vi "CCarga_LVDT_Actuador.vi"() -> ()   [LabVIEW 2015]
uses:
  <vilib>/Utility/file.llb/Read Delimited Spreadsheet (DBL).vi
  variables offset.vi
panel:
  in  "Instrucciones":bool
  out "LVDT RAW":dbl
  out "LVDT":dbl
  out "vector poros":dbl[](array[numeric]) format="%.2f"
  out "C_Poros":dbl
  out "P_Poros":dbl
  out "Poros":dbl
  out "offset 9":dbl
  in  "SAVE":bool
  in  "Tiempo \nMuestreo":dbl=3.0 format="%#_13g"
  out "READ!":bool
  in  "BttActuador":bool
  out "Boolean":bool
  out "offset 8":dbl
  out "offset 7":dbl
  in  "offsets":bool
  out "C_Celda":dbl
  out "C_lvdt":dbl
  out "P_Celda":dbl
  out "P_lvdt":dbl
  out "all rows":dbl[][](array[numeric])
  out "vector carga":dbl[](array[numeric]) format="%.2f"
  out "vector desp":dbl[](array[numeric]) format="%.2f"
  out "Carga":dbl
  in  "Tab Control":enum32{"SENSORES"}(tab)
  out "Waveform Celda de Carga":dynamicdata(graph)
  out "Waveform LVDT":dynamicdata(graph)
  out "LOAD RAW":dbl
  out "Waveform Presión de Poros":dynamicdata(graph)
  out "TIME SEC":dbl[](array[numeric]) format="%.2f"
  out "x/y":dbl
  out "Boolean 2":bool
  out "tiempo [min]":ext
  out "path":path
  in  "stop":bool
  in  "Conect":bool
  in  "Filename":path=path "Ensayo_Dyn_M"
  # "Seg."
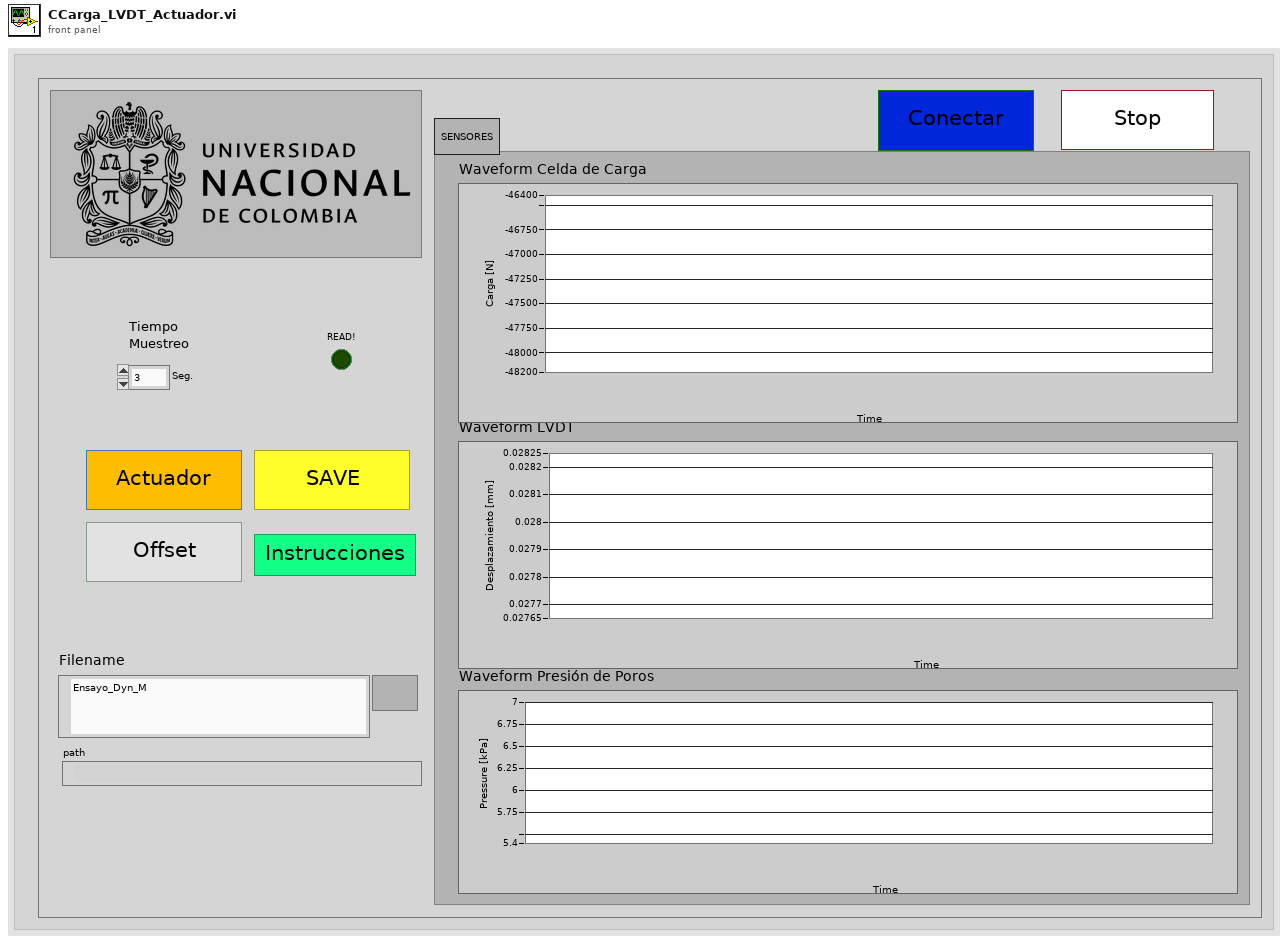
[diagram p1: front panel]
types:
  T1 = enum16{"open", "open or create", "create or replace", "create", "open (read-only)"}
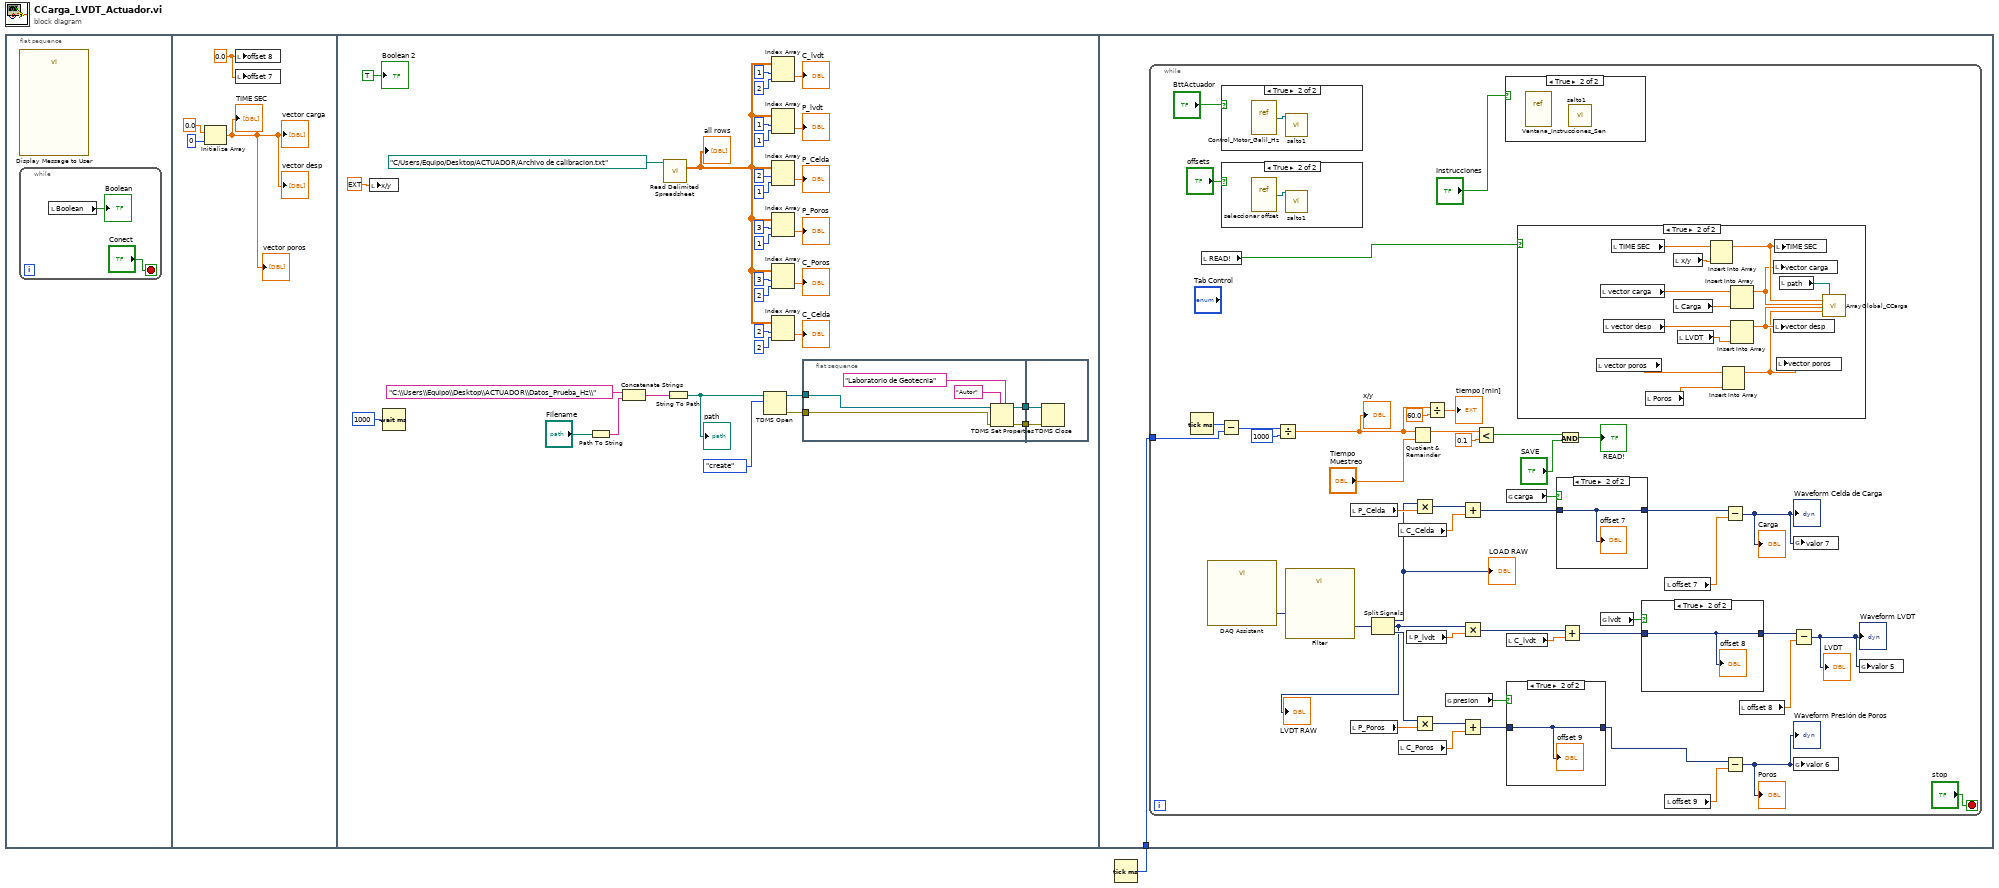
[diagram p0: block diagram]
diagram:
  n1 = flat-sequence {
    tunnel: w1 -> [w49]
    frame #0 {
      n2 = call "Display Message to User"() -> ()  [unwired: 10 in, 2 out]
      n3 = while {
        stop <- "Conect" stop-if-true
        n4 = local read "Boolean"() -> (→"Boolean":bool)
      }
    }
    frame #1 {
      w5 = 0.0
      n5 = Initialize Array(0.0, 0 ("dimension size")) -> (→"TIME SEC" →"vector desp" →"vector carga" →"vector poros":dbl[])
      n6 = local write "offset 8"(w5) -> ()
      n7 = local write "offset 7"(w5) -> ()
    }
    frame #2 {
      n8 = local write "x/y"(ext 0.0 ("x-y*floor(x/y)")) -> ()
      n9 = Wait (ms)(milliseconds to wait=u32 1000) -> ()  [unwired: 1 out]
      n10 = Path To String(path="Filename") -> (string=w37:string)
      n11 = Concatenate Strings("C:\\Users\\Equipo\\Desktop\\ACTUADOR\\Datos_Prueba_Hz\\", w37) -> (w36:string)
      n12 = call-poly <vilib>:"Read Delimited Spreadsheet.vi"("file path (dialog if empty)"=path "C:/Users/Equipo/Desktop/ACTUADOR/Archivo de calibracion.txt") -> ("all rows"=w8:dbl[][])  [unwired: 9 in, 5 out]
      "all rows" <- w8
      n13 = String To Path(string=w36) -> (path=w34:path)
      "path" <- w34
      n14 = TDMS Open(10:T1."create" ("operation (0:open)"), 11:w34) -> (0:w30:errorcluster, 3:w31:refnum<k34>)  [unwired: 5 in]
      n15 = Index Array(array=w8, index (row)=1, index (col)=2 ("disabled index (col)")) -> (element=→"C_lvdt":dbl)
      n16 = Index Array(array=w8, index (row)=1, index (col)=1 ("disabled index (col)")) -> (element=→"P_lvdt":dbl)
      n17 = Index Array(array=w8, index (row)=2, index (col)=1 ("disabled index (col)")) -> (element=→"P_Celda":dbl)
      n18 = Index Array(array=w8, index (row)=3, index (col)=1 ("disabled index (col)")) -> (element=→"P_Poros":dbl)
      n19 = Index Array(array=w8, index (row)=3, index (col)=2 ("disabled index (col)")) -> (element=→"C_Poros":dbl)
      n20 = Index Array(array=w8, index (row)=2, index (col)=2 ("disabled index (col)")) -> (element=→"C_Celda":dbl)
      n21 = flat-sequence {
        tunnel: [w44] -> w39
        tunnel: [w43] -> w38
        tunnel: w31 -> [w42]
        tunnel: w30 -> [w41]
        tunnel: w39 -> [w48]
        tunnel: w38 -> [w47]
        frame #0 {
          n22 = TDMS Set Properties(5:"Laboratorio de Geotecnia" ("property name"), 7:"Autor" ("property name"), 8:w41, 11:w42) -> (0:w43:errorcluster, 3:w44:refnum<k34>)  [unwired: 2 in, 2 out]
        }
        frame #1 {
          n23 = TDMS Close(8:w47, 11:w48) -> ()  [unwired: 2 out]
        }
      }
      "Boolean 2" <- TRUE
    }
    frame #3 {
      n24 = while {
        tunnel: w49 -> [w90]
        stop <- "stop" stop-if-true
        n25 = Tick Count (ms)() -> (millisecond timer value=w95:u32)
        n26 = local read "READ!"() -> (w72:bool)
        n27 = call "DAQ Assistant"() -> ("data"=w66:dynamicdata)  [unwired: 16 in, 3 out]
        n28 = Subtract(x=w95, y=w90) -> (x-y=w94:u32)
        n29 = case shown="True" "BttActuador" {
          frame False {
          }
          frame True {
            n30 = vi-ref "Control_Motor_Galil_Hz.vi"() -> (w112:refnum<vi>)
            n31 = call "salto1.vi"("reference"=w112) -> ()  [unwired: 15 in]
          }
        }
        n32 = case shown="True" "offsets" {
          frame False {
          }
          frame True {
            n33 = vi-ref "seleccionar offset.vi"() -> (w113:refnum<vi>)
            n34 = call "salto1.vi"("reference"=w113) -> ()  [unwired: 15 in]
          }
        }
        n35 = Divide(x=w94, y=u32 1000) -> (x/y=w75:dbl)
        "x/y" <- w75
        n36 = call "Filter"("Signal"=w66) -> ("Filtered Signal"=w65:dynamicdata)  [unwired: 9 in, 1 out]
        n37 = local read "P_Celda"() -> (w81:dbl)
        n38 = local read "P_Poros"() -> (w58:dbl)
        n39 = Split Signals(w65) -> (w51:dynamicdata, w52:dynamicdata, w61:dynamicdata)  [unwired: 3 in]
        "LVDT RAW" <- w52
        "LOAD RAW" <- w51
        n40 = local read "C_Celda"() -> (w80:dbl)
        n41 = local read "C_Poros"() -> (w57:dbl)
        n42 = local read "P_lvdt"() -> (w70:dbl)
        n43 = Quotient & Remainder(x=w75, y="Tiempo \nMuestreo") -> (x-y*floor(x/y)=w76:dbl)  [unwired: 1 out]
        n44 = Multiply(x=w51, y=w81) -> (x*y=w79:dynamicdata)
        n45 = Multiply(x=w61, y=w58) -> (x*y=w60:dynamicdata)
        n46 = Divide(x=w75, y=60.0) -> (x/y=→"tiempo [min]":dbl)
        n47 = global read "variables offset.vi" "presion"() -> (w55:bool)
        n48 = Add(x=w79, y=w80) -> (x+y=w78:dynamicdata)
        n49 = Multiply(x=w52, y=w70) -> (x*y=w71:dynamicdata)
        n50 = Add(x=w60, y=w57) -> (x+y=w59:dynamicdata)
        n51 = Less?(x=w76, y=0.1) -> (x < y?=w63:bool)
        n52 = case shown="True" "Instrucciones" {
          frame False {
          }
          frame True {
            n53 = vi-ref "Ventana_Instrucciones_Sen.vi"() -> ()  [unwired: 1 out]
            n54 = call "salto1.vi"() -> ()  [unwired: 16 in]
          }
        }
        n55 = global read "variables offset.vi" "carga"() -> (w85:bool)
        n56 = local read "C_lvdt"() -> (w69:dbl)
        n57 = case shown="True" w55 {
          tunnel: [w97 w98] -> w53
          tunnel: w59 -> [w97 w98]
          frame False {
          }
          frame True {
            "offset 9" <- w98
          }
        }
        n58 = case shown="True" w72 {
          frame False {
          }
          frame True {
            n59 = local read "vector poros"() -> (w101:dbl[])
            n60 = local read "vector carga"() -> (w109:dbl[])
            n61 = local read "vector desp"() -> (w107:dbl[])
            n62 = local read "TIME SEC"() -> (w111:dbl[])
            n63 = local read "Poros"() -> (w100:dbl)
            n64 = local read "x/y"() -> (w110:dbl)
            n65 = local read "Carga"() -> (w108:dbl)
            n66 = local read "LVDT"() -> (w106:dbl)
            n67 = Insert Into Array(array=w111, new element=w110) -> (w105:dbl[])  [unwired: 1 in]
            n68 = Insert Into Array(array=w101, new element=w100) -> (w99:dbl[])  [unwired: 1 in]
            n69 = Insert Into Array(array=w109, new element=w108) -> (w104:dbl[])  [unwired: 1 in]
            n70 = Insert Into Array(array=w107, new element=w106) -> (w103:dbl[])  [unwired: 1 in]
            n71 = local write "vector carga"(w104) -> ()
            n72 = local write "vector desp"(w103) -> ()
            n73 = local write "TIME SEC"(w105) -> ()
            n74 = local write "vector poros"(w99) -> ()
            n75 = local read "path"() -> (w102:path)
            n76 = call "ArrayGlobal_CCarga.vi"("Tiempo"=w105, "Carga"=w104, "LVDT"=w103, "Pres_Poros"=w99, "Path"=w102) -> ()  [unwired: 14 in, 1 out]
          }
        }
        n77 = case shown="True" w85 {
          tunnel: w78 -> [w116 w117]
          tunnel: [w116 w117] -> w86
          frame False {
          }
          frame True {
            "offset 7" <- w117
          }
        }
        n78 = And(x=w63, y="SAVE") -> (x .and. y?=→"READ!":bool)
        n79 = Add(x=w71, y=w69) -> (x+y=w68:dynamicdata)
        n80 = global read "variables offset.vi" "lvdt"() -> (w84:bool)
        n81 = case shown="True" w84 {
          tunnel: [w114 w115] -> w87
          tunnel: w68 -> [w114 w115]
          frame False {
          }
          frame True {
            "offset 8" <- w115
          }
        }
        n82 = local read "offset 7"() -> (w89:dbl)
        n83 = local read "offset 9"() -> (w56:dbl)
        n84 = Subtract(x=w86, y=w89) -> (x-y=w74:dynamicdata)
        "Carga" <- w74
        "Waveform Celda de Carga" <- w74
        n85 = Subtract(x=w53, y=w56) -> (x-y=w54:dynamicdata)
        "Poros" <- w54
        "Waveform Presión de Poros" <- w54
        n86 = local read "offset 8"() -> (w88:dbl)
        n87 = Subtract(x=w87, y=w88) -> (x-y=w73:dynamicdata)
        "LVDT" <- w73
        "Waveform LVDT" <- w73
        n88 = global write "variables offset.vi" "valor 7"(w74) -> ()
        n89 = global write "variables offset.vi" "valor 6"(w54) -> ()
        n90 = global write "variables offset.vi" "valor 5"(w73) -> ()
      }
    }
  }
  n91 = Tick Count (ms)() -> (millisecond timer value=w1:u32)
